vi "Set Timeout.vi"(8 "error in (no error)":errorcluster, 10 "Timeout (ms)":i32, 11 "JKI SM in":refnum<class "JKI SM.lvclass">) -> (0 "error out":errorcluster, 3 "JKI SM out":refnum<class "JKI SM.lvclass">)   [LabVIEW 2020, in "JKI State Machine API.lvlib" / "JKI SM.lvclass"]
uses:
  JKI SM.lvclass
  JKI SM.lvclass/JKI SM.ctl
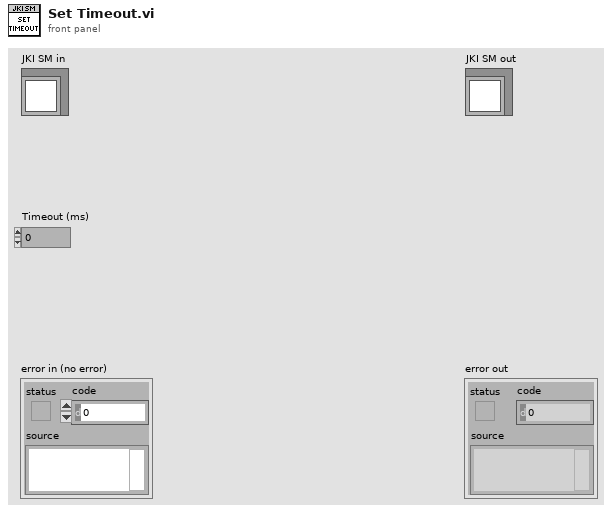
[diagram p1: front panel]
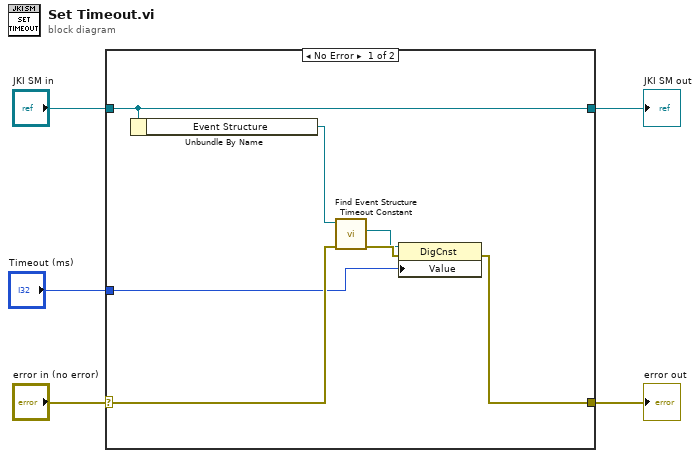
[diagram p0: block diagram]
diagram:
  n1 = case shown="No Error" "error in (no error)" {
    selector: "error in (no error)" -> [w10 w14]
    tunnel: [w8 w14] -> w4
    tunnel: [w12 w13] -> w2
    tunnel: "JKI SM in" -> [w12 w13]
    tunnel: "Timeout (ms)" -> [w6 _]
    frame No Error {
      n2 = Unbundle By Name(w12) -> ("Event Structure"=w11:refnum<vi>)
      n3 = call "Find Event Structure Timeout Constant.vi"("error in (no error)"=w10, "EventStructure in"=w11) -> ("error out"=w9:errorcluster, "DigitalNumericConstant out"=w7:refnum<vi>)  [unwired: 8 in]
      n4 = property class="DigCnst"(reference=w7, error in=w9, "Value"=w6) -> (error out=w8:errorcluster)  [unwired: 1 out]
    }
    frame Error {
    }
  }
  "error out" <- w4
  "JKI SM out" <- w2
